vi "DAQ - 45 Modules - SubVI.vi"(11 "array":dbl[](array[numeric])) -> (3 "output array":dbl[](array[numeric]))   [LabVIEW 2013]
panel:
  out "voltage (V)":dbl
  out "error out":errorcluster
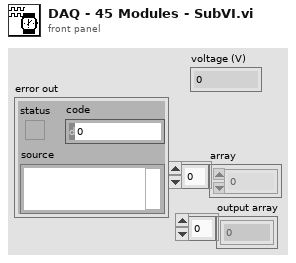
[diagram p1: front panel]
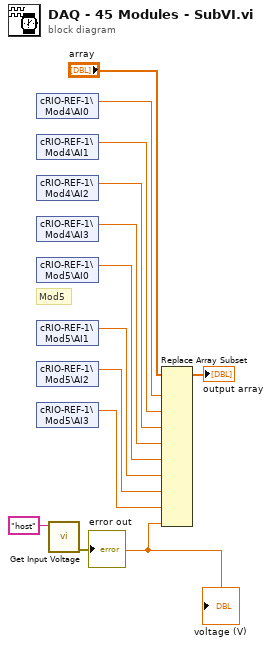
[diagram p0: block diagram]
diagram:
  # "Mod5"
  n1 = shared-variable "cRIO-REF-1\\Mod4\\AI0"() -> (w7:dbl)  [unwired: 1 in, 1 out]
  n2 = shared-variable "cRIO-REF-1\\Mod4\\AI1"() -> (w6:dbl)  [unwired: 1 in, 1 out]
  n3 = shared-variable "cRIO-REF-1\\Mod4\\AI2"() -> (w5:dbl)  [unwired: 1 in, 1 out]
  n4 = shared-variable "cRIO-REF-1\\Mod4\\AI3"() -> (w4:dbl)  [unwired: 1 in, 1 out]
  n5 = shared-variable "cRIO-REF-1\\Mod5\\AI0"() -> (w13:dbl)  [unwired: 1 in, 1 out]
  n6 = shared-variable "cRIO-REF-1\\Mod5\\AI1"() -> (w12:dbl)  [unwired: 1 in, 1 out]
  n7 = shared-variable "cRIO-REF-1\\Mod5\\AI2"() -> (w11:dbl)  [unwired: 1 in, 1 out]
  n8 = shared-variable "cRIO-REF-1\\Mod5\\AI3"() -> (w10:dbl)  [unwired: 1 in, 1 out]
  n9 = call "Get Input Voltage.vi"("host address (host)"="host") -> ("error out"=→"error out":errorcluster, "voltage (V)"=w1:dbl)  [unwired: 1 in, 8 out]
  "voltage (V)" <- w1
  n10 = Replace Array Subset(array="array", new element #1=w7, new element #2=w6, new element #3=w5, new element #4=w4, new element #5=w13, new element #6=w12, new element #7=w11, new element #8=w10, new element #9=w1) -> (→"output array":dbl[])  [unwired: 9 in]
